vi "Control Experiment Class from JSON.vi"(8 "error in (no error)":errorcluster, 10 "JSON":string, 11 "Control Experiment in":refnum<class "Control Experiment.lvclass">) -> (0 "error out":errorcluster, 3 "Control Experiment out":refnum<class "Control Experiment.lvclass">)   [LabVIEW 2019, in "Control Experiment.lvclass"]
uses:
  Control Experiment.lvclass
  Control Experiment.lvclass/Control Experiment.ctl
  <userlib>/LevyLab/Instrument Framework/SMOs/Instrument/Instrument.lvclass
  <userlib>/LevyLab/Instrument Framework/SMOs/Instrument/Instrument.lvclass/Instrument.ctl
  dbafe0ef-e718-4924-8c3c-ddc720cb6ca1.vi
  <vilib>/JDP Science/JSONtext/JSON text to Variant.vi
  <vilib>/JDP Science/JSONtext/LVClass Serializer/JSONtext LVClass Serializer.lvclass
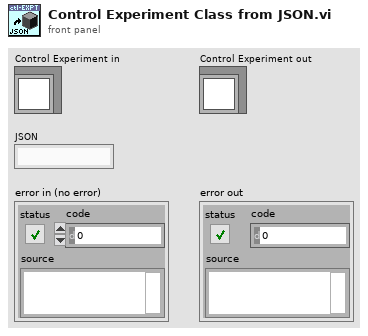
[diagram p1: front panel]
types:
  T1 = typedef "Control Experiment.lvclass/Experiment Description--cluster.ctl" = cluster{"User":string, "Device":string, "Device Path":path, "Device Description":string, "Experiment Path":path, "Experiment Description":string, "Instrument":T2, "Instruments":cluster{"class path":path, "Address":string, "Type":T3}[], "Sweep":cluster{"key":string, "value":variant}[]}
  T2 = typedef "Control Experiment.lvclass/Instrument--enum.ctl" = enum16{"----- AFM/EBL -----", "AGILENT", "CYPHER", "Gemini2", "JEOL", "MFP3D", "----- Cryostat -----", "CF900", "DR200", "MNK", "PPMS (simulated)", "PPMS 1", "PPMS 2", "PPMS 3", "----- Optics -----", "THz 1 (Element 2/Montana)", "THz 2 (Tsunami/Janis)"}
  T3 = typedef "Control Experiment.lvclass/Instrument Types--combo.ctl" = string
  T4 = typedef "Control Experiment.lvclass/Wiring Description--cluster.ctl" = cluster{"Lockin Ch":i32[], "KH":cluster{"Electrodes":string[], "Labels":string[]}, "not KH":cluster{"Electrodes":string[], "Labels":string[]}}
  T5 = cluster{"json":string, "Experiment":T1, "Wiring Configuration":T4}
  T6 = cluster{"class path":path, "Address":string, "Type":T3}[]
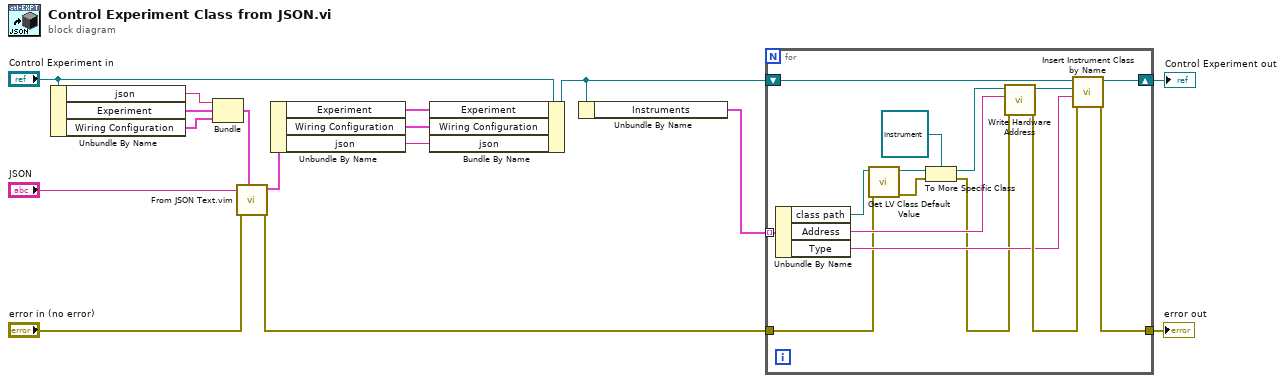
[diagram p0: block diagram]
diagram:
  n1 = Unbundle By Name("Control Experiment in") -> ("json"=w2:string, "Experiment"=w11:T1, "Wiring Configuration"=w10:T4)
  n2 = Bundle("json"=w2, "Experiment"=w11, "Wiring Configuration"=w10) -> (w9:T5)  [unwired: 1 in]
  n3 = call "From JSON Text.vim"("Data Type and Default Value"=w9, "error in (no error)"="error in (no error)", "JSON"="JSON") -> ("error out"=w13:errorcluster, "Data out"=w5:T5)  [unwired: 7 in]
  n4 = Unbundle By Name(w5) -> ("Experiment"=w8:T1, "Wiring Configuration"=w7:T4, "json"=w1:string)
  n5 = Bundle By Name(cluster="Control Experiment in", "Experiment"=w8, "Wiring Configuration"=w7, "json"=w1) -> (w4:refnum<class "Control Experiment.lvclass">)
  n6 = Unbundle By Name(w4) -> ("Instruments"=w3:T6)
  n7 = for {
    tunnel: w3 -> [w31] mode=indexing
    tunnel: w13 -> [w19]
    tunnel: [w22] -> w15
    shift-right: [w25] -> w6
    shift-left: w4 -> [w26]
    n8 = Unbundle By Name(w31) -> ("class path"=w18:path, "Address"=w21:string, "Type"=w20:T3)
    n9 = call <vilib>:"Get LV Class Default Value.vi"("error in (no error)"=w19, "class path"=w18) -> ("error out"=w28:errorcluster, "object"=w30:refnum<class>)  [unwired: 8 in]
    n10 = To More Specific Class(target class=refnum<class "Instrument.lvclass"> refnum ("Instrument in"), reference=w30, error in=w28) -> (specific class reference=w27:refnum<class "Instrument.lvclass">, error out=w17:errorcluster)
    n11 = call <userlib>:"Write Hardware Address.vi"("error in (no error)"=w17, "Address"=w21, "Instrument in"=w27) -> ("error out"=w23:errorcluster, "Instrument out"=w24:refnum<class "Instrument.lvclass">)  [unwired: 7 in]
    n12 = call "Insert Instrument Class by Name.vi"("error in (no error)"=w23, "Type"=w20, "Instrument in"=w24, "Control Experiment in"=w26) -> ("error out"=w22:errorcluster, "Control Experiment out"=w25:refnum<class "Control Experiment.lvclass">)  [unwired: 4 in, 2 out]
  }
  "Control Experiment out" <- w6
  "error out" <- w15
